vi "Delete Group.vi"(0 "Node Ptr":T1 format="%.0x") -> ()   [LabVIEW 2024, in "Embedded TDMS Logger System Explorer.lvlib"]
doc: "Deletes the user selected (by right click on the item) group section in the System Definition of the Custom Device."
uses:
  Embedded TDMS Logger System Explorer.lvlib
  <vilib>/NI VeriStand/Custom Device API/Custom Device Item Ref.ctl
  <vilib>/NI VeriStand/Custom Device API/Custom Device API.lvlib
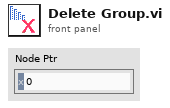
[diagram p1: front panel]
types:
  T1 = typedef "Custom Device API.lvlib/Custom Device Item Ref.ctl" = u64
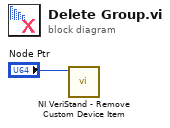
[diagram p0: block diagram]
diagram:
  n1 = call <vilib>:"NI VeriStand - Remove Custom Device Item.vi"("Item Ref in"="Node Ptr") -> ()  [unwired: 9 in, 2 out]
